vi "Command Loop.vi"(8 "Error in":errorcluster, 10 "Queue Refs":T1, 11 "Device Reference in":T2 format="%.0x") -> ()   [LabVIEW 2025, in "Runtime Configuration Support Example Engine.lvlib"]
uses:
  Runtime Configuration Support Example Engine.lvlib
  <vilib>/NI VeriStand/Custom Device API/Custom Device Item Ref.ctl
  Shared/Compiled.Settings.ctl
  <vilib>/NI VeriStand/Custom Device API/Message Response (String).ctl
  <vilib>/NI VeriStand/Custom Device API/Message Response (Byte Array).ctl
  <vilib>/NI VeriStand/Custom Device API/Custom Device API.lvlib
  Shared/Runtime Configuration Support Example Shared.lvlib
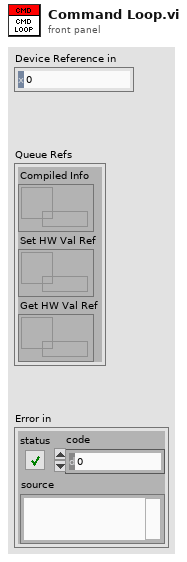
[diagram p1: front panel]
types:
  T1 = cluster{"Compiled Info":refnum<queue>, "Set HW Val Ref":refnum<queue>, "Get HW Val Ref":refnum<queue>}
  T2 = typedef "Custom Device API.lvlib/Custom Device Item Ref.ctl" = u64
  T3 = typedef "Custom Device API.lvlib/Custom Device Engine Event Ref.ctl" = refnum<event-registration>
  T4 = typedef "Custom Device API.lvlib/Message Response (String).ctl" = cluster{"Response":string, "Error":errorcluster}
  T5 = typedef "Custom Device API.lvlib/Message Response (Byte Array).ctl" = cluster{"Response":u8[], "Error":errorcluster}
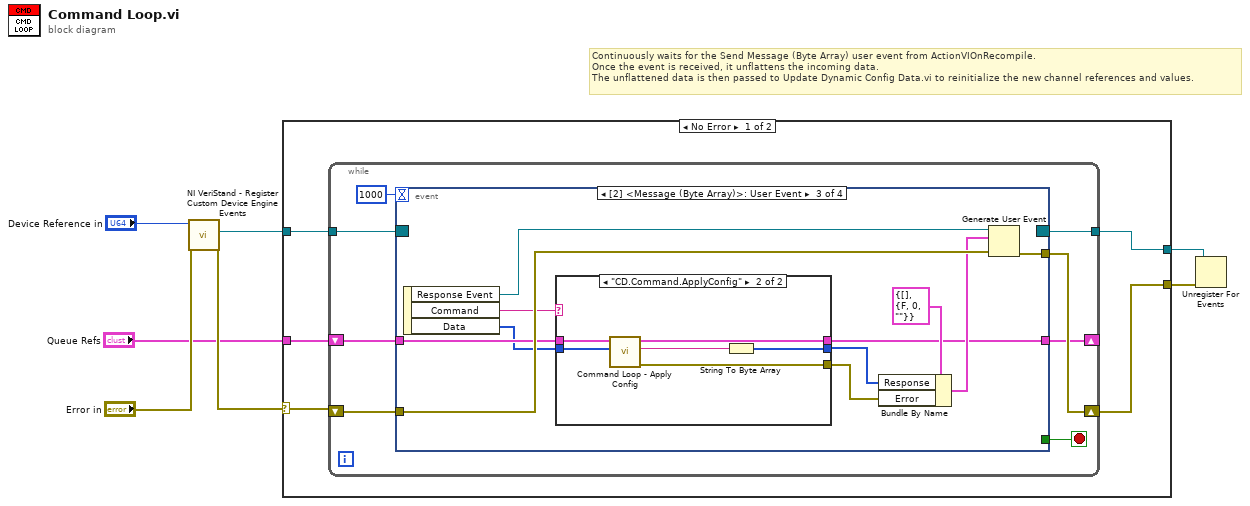
[diagram p0: block diagram]
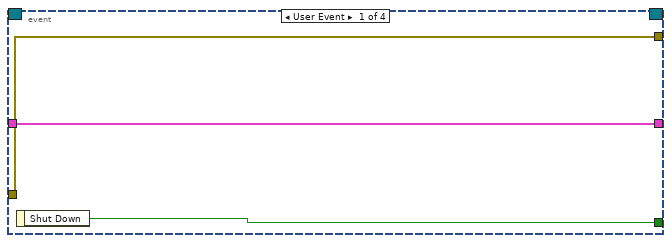
[diagram p2: hidden frame]
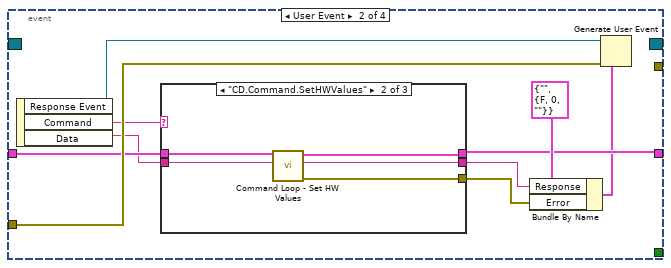
[diagram p3: hidden frame]
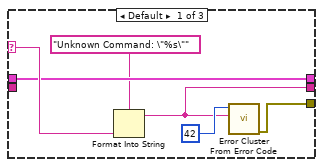
[diagram p4: hidden frame]
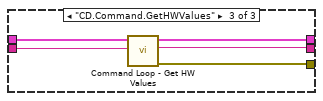
[diagram p5: hidden frame]
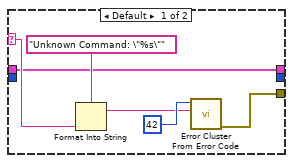
[diagram p6: hidden frame]
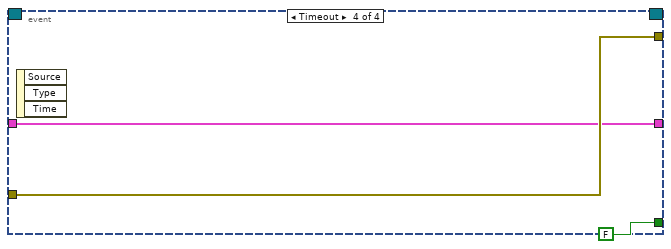
[diagram p7: hidden frame]
diagram:
  # "Continuously waits for the Send Message (Byte Array) user event from ActionVIOnRecompile.\nOnce the event is received, it unflattens the incoming data.\nThe unflattened data is then passed to Update Dynamic Config Data.vi to reinitialize the new channel references and values."
  n1 = call <vilib>:"NI VeriStand - Register Custom Device Engine Events.vi"("error in (no error)"="Error in", "Device Ref in"="Device Reference in") -> ("error out"=w5:errorcluster, "Custom Device Engine Event Ref"=w2:T3)  [unwired: 7 in, 1 out]
  n2 = case shown="No Error" w5 {
    selector: w5 -> [w12 w76]
    tunnel: [w10 _] -> w4
    tunnel: [w11 w76] -> w7
    tunnel: w2 -> [w9 _]
    tunnel: "Queue Refs" -> [w8 _]
    frame No Error {
      n3 = while {
        tunnel: [w17] -> w10
        shift-right: [w19] -> w11
        shift-left: w12 -> [w20]
        tunnel: w9 -> [w16]
        shift-right: [w13] -> _
        shift-left: w8 -> [w14]
        stop <- w18 stop-if-true
        n4 = event shown="[2] <Message (Byte Array)>: User Event" {
          selector: w16 -> [_ _ _ _]
          dyn-events: [_ _ _ _] -> w17
          timeout: 1000 -> [_ _ _ _]
          tunnel: [w22 _ _ FALSE ("Shut Down")] -> w18
          tunnel: [w23 _ w58 w75] -> w19
          tunnel: w20 -> [w23 w33 w59 w75]
          tunnel: w14 -> [w21 w28 w52 w73]
          tunnel: [w21 w27 w51 w73] -> w13
          event User Event {
            n5 = event-data() -> ("Shut Down"=w22:bool)  [unwired: 1 in]
          }
          event User Event {
            n6 = event-data() -> ("Response Event"=w29:refnum<user-event>, "Command"=w30:string, "Data"=w26:string)  [unwired: 1 in]
            n7 = case shown="\"CD.Command.SetHWValues\"" w30 {
              selector: w30 -> [w37 _ _]
              tunnel: w28 -> [w36 w40 w48]
              tunnel: [w36 w43 w46] -> w27
              tunnel: w26 -> [_ w42 w47]
              tunnel: [w34 w41 w45] -> w24
              tunnel: [w39 w44 w49] -> w32
              frame Default {
                n8 = Format Into String(format string="Unknown Command: \"%s\"", w37) -> (resulting string=w34:string)  [unwired: 2 in, 1 out]
                n9 = call <vilib>:"Error Cluster From Error Code.vi"("error message (\"\")"=w34, "error code (0)"=42) -> ("error out"=w39:errorcluster)  [unwired: 7 in]
              }
              frame "CD.Command.SetHWValues" {
                n10 = call "Command Loop - Set HW Values.vi"("Data"=w42, "Queue Refs in"=w40) -> ("error out"=w44:errorcluster, "Response"=w41:string, "Queue Refs out"=w43:T1)  [unwired: 7 in]
              }
              frame "CD.Command.GetHWValues" {
                n11 = call "Command Loop - Get HW Values.vi"("Data"=w47, "Queue Refs in"=w48) -> ("error out"=w49:errorcluster, "Response"=w45:string, "Queue Refs out"=w46:T1)  [unwired: 7 in]
              }
            }
            n12 = Bundle By Name(cluster=T4 {"Response"="", "Error"={"status"=FALSE, "code"=0, "source"=""}} ("event data"), "Response"=w24, "Error"=w32) -> (w25:T4)
            n13 = Generate User Event(user event=w29, event data cluster=w25, error in=w33) -> ()  [unwired: 1 in, 2 out]
          }
          event User Event {
            n14 = event-data() -> ("Response Event"=w57:refnum<user-event>, "Command"=w53:string, "Data"=w50:u8[])  [unwired: 1 in]
            n15 = case shown="\"CD.Command.ApplyConfig\"" w53 {
              selector: w53 -> [w63 _]
              tunnel: [w66 w72] -> w60
              tunnel: [_ w70] -> w55
              tunnel: w52 -> [w61 w68]
              tunnel: [w61 w67] -> w51
              tunnel: w50 -> [_ w71]
              frame Default {
                n16 = Format Into String(format string="Unknown Command: \"%s\"", w63) -> (resulting string=w62:string)  [unwired: 2 in, 1 out]
                n17 = call <vilib>:"Error Cluster From Error Code.vi"("error message (\"\")"=w62, "error code (0)"=42) -> ("error out"=w66:errorcluster)  [unwired: 7 in]
              }
              frame "CD.Command.ApplyConfig" {
                n18 = call "Command Loop - Apply Config.vi"("Data"=w71, "Queue Refs in"=w68) -> ("error out"=w72:errorcluster, "Response"=w69:string, "Queue Refs out"=w67:T1)  [unwired: 7 in]
                n19 = String To Byte Array(string=w69) -> (unsigned byte array=w70:u8[])
              }
            }
            n20 = Bundle By Name(cluster=T5 {"Response"=[], "Error"={"status"=FALSE, "code"=0, "source"=""}} ("event data"), "Response"=w55, "Error"=w60) -> (w54:T5)
            n21 = Generate User Event(user event=w57, event data cluster=w54, error in=w59) -> (error out=w58:errorcluster)  [unwired: 1 in, 1 out]
          }
          event Timeout {
            n22 = event-data() -> ()  [unwired: 1 in, 3 out]
          }
        }
      }
    }
    frame Error {
    }
  }
  n23 = Unregister For Events(event registration refnum=w4, error in=w7) -> ()  [unwired: 1 out]
